vi "writeToXML.vi"(8 "error in (no error)":errorcluster, 10 "ClassLabel":string, 11 "OffsetCommands in":refnum<class "OffsetCommands.lvclass">) -> (0 "error out":errorcluster, 2 "XML out":string, 3 "OffsetCommands out":refnum<class "OffsetCommands.lvclass">)   [LabVIEW 2022 SP3, in "TCSDataDefinitions.lvlib" / "TCSCommand.lvlib" / "OffsetCommands.lvlib" / "OffsetCommands.lvclass"]
uses:
  OffsetCommands.lvclass
  TCSTcsCommand/TCSTcsCommand.lvclass
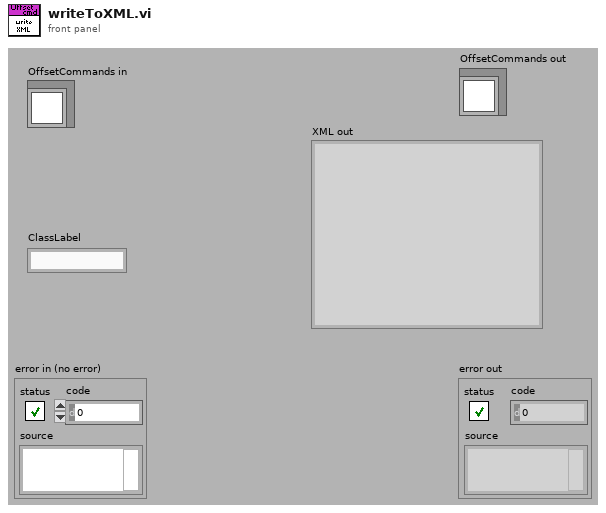
[diagram p1: front panel]
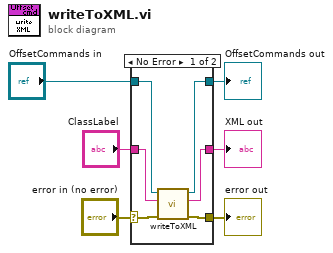
[diagram p0: block diagram]
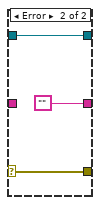
[diagram p2: hidden frame]
diagram:
  n1 = case shown="No Error" "error in (no error)" {
    selector: "error in (no error)" -> [w8 w15]
    tunnel: [w7 w15] -> w5
    tunnel: [w10 w14] -> w4
    tunnel: "OffsetCommands in" -> [w11 w14]
    tunnel: "ClassLabel" -> [w12 _]
    tunnel: [w9 ""] -> w2
    frame No Error {
      n2 = call-parent "writeToXML.vi"("error in (no error)"=w8, "ClassLabel"=w12, "TCSTcsCommand in"=w11) -> ("error out"=w7:errorcluster, "XML out"=w9:string, "TCSTcsCommand out"=w10:refnum<class "OffsetCommands.lvclass">)  [unwired: 6 in]
    }
    frame Error {
    }
  }
  "error out" <- w5
  "OffsetCommands out" <- w4
  "XML out" <- w2
